vi "TEST - Periodic Trigger.vi"(8 "error in (no error)":errorcluster) -> (0 "error out":errorcluster, 2 "pass":bool)   [LabVIEW 2020]
uses:
  <userlib>/_OpenG.lib/error/error.llb/openg_error.lvlib
  source/library/openg_time.lvlib
panel:
  out "sum":i16
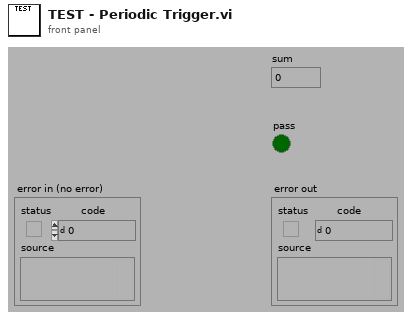
[diagram p1: front panel]
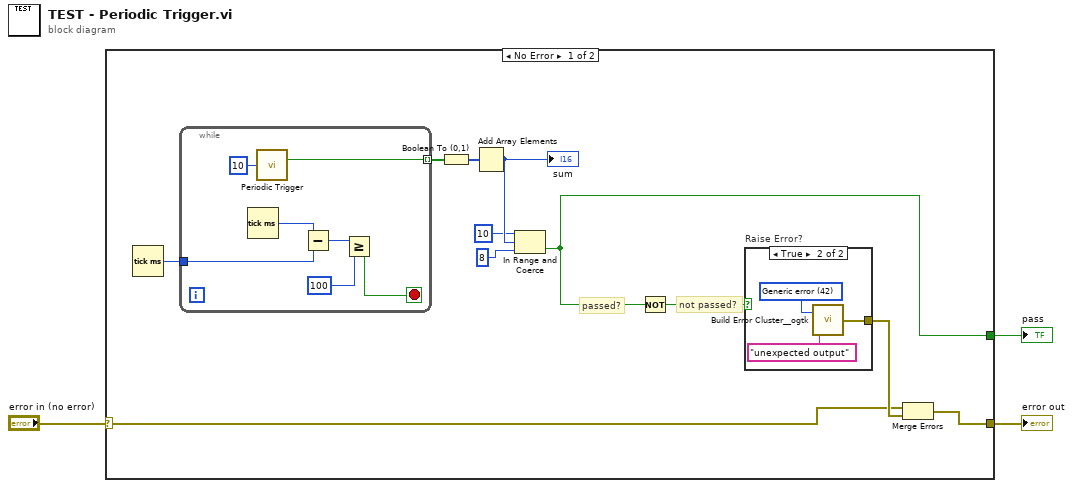
[diagram p0: block diagram]
diagram:
  n1 = case shown="No Error" "error in (no error)" {
    selector: "error in (no error)" -> [w8 w25]
    tunnel: [w4 _] -> w3
    tunnel: [w14 w25] -> w1
    frame No Error {
      # "not passed?"
      # "passed?"
      n2 = Tick Count (ms)() -> (millisecond timer value=w11:u32)
      n3 = while {
        tunnel: w11 -> [w19]
        tunnel: [w20] -> w10 mode=indexing
        stop <- w16 stop-if-true
        n4 = Tick Count (ms)() -> (millisecond timer value=w15:u32)
        n5 = call "Periodic Trigger.vi"("time (ms)"=u32 10) -> ("Triggered"=w20:bool)  [unwired: 12 in, 2 out]
        n6 = Subtract(x=w15, y=w19) -> (x-y=w18:u32)
        n7 = Greater Or Equal?(x=w18, y=u32 100) -> (x >= y?=w16:bool)
      }
      n8 = Boolean To (0,1)(Boolean=w10) -> (0, 1=w9:i16[])
      n9 = Add Array Elements(numeric array=w9) -> (sum=w7:i16)
      "sum" <- w7
      n10 = In Range and Coerce(upper limit=i16 10 ("sum"), x=w7, lower limit=i16 8 ("sum")) -> (In Range?=w4:bool)  [unwired: 1 out]
      n11 = Not(x=w4) -> (.not. x?=w12:bool)
      n12 = case "Raise Error?" shown="True" w12 {
        tunnel: [_ w22] -> w13
        frame False {
        }
        frame True {
          w23 = 42 items=["No error", "Argument error", "Memory is full", "Out of zone", "End of file", "File already open", "Generic file I/O error", "File not found", "File permission error", "Disk is full", "Duplicate path", "Too many files open", "System feature not enabled", "Resource file not found", "Cannot add resource", "Resource not found", "Image not found", "Image memory error", "Pen does not exist", "Config type invalid", "Config token not found", "Config parse error", "Config memory error", "Bad external code format", "Bad external code offset", "External code not present", "Null window", "Destroy window error", "Null menu", "Print aborted", "Bad print record", "Print driver error", "Windows error during printing", "Memory error during printing", "Print dialog error", "Generic print error", "Invalid device refnum", "Device not found", "Device parameter error", "Device unit error", "Cannot open device", "Device call aborted", "Generic error", "Cancelled by user", "Object ID too low", "Object ID too high", "Object not in heap", "Unknown heap", "Unknown object (invalid DefProc)", "Unknown object (DefProc not in table)", "Message out of range", "Invalid (null) method", "Unknown message", "Manager call not supported", "Bad address", "Network operation in progress", "Network operation timed out", "Connection is busy", "Network attribute not supported", "Network error", "Address in use", "System out of memory", "Connection aborted", "Connection refused", "Not connected", "Already connected", "Connection closed", "Initialization error (interapplication manager)", "Bad occurrence", "Wait on unbound occurrence handler", "Occurrence queue overflow", "Datalog type conflict", "Unused", "Unrecognized type (interapplication manager)", "Memory corrupt", "Failed to make temporary DLL", "Old CIN version", "Drag socket not found", "Failed to load drop-object", "Failed to register OLE object", "Failed to release OLE object", "Format specifier type mismatch", "Unknown format specifier", "Too few format specifiers", "Too many format specifiers", "Scan failed", "Newer CIN version", "Error converting to variant", "Runtime menu error", "Password tampered", "Variant attribute not found", "Incompatible variant data type", "Event data is not available", "Event Store is not present", "Occurrence is not found", "Event Queue is not created", "Event info is not available", "Refnum passed is NULL", "Error retrieving Class GUID", "Error retrieving CoClass GUID", "Error retrieving TypeLib GUID.", "Bad built application magic bytes.", "Specific driver is different from the specific driver associated with the Logical Name.", "There is no session opened to the class driver.", "Max Error", "MAX - Error with config objects", "MAX - Error loading configuration", "MAX - Group not supported"]
          n13 = call <userlib>:"Build Error Cluster__ogtk.vi"("String to Prepend to source (\"\")"="unexpected output" ("String to Prepend to source (\"\")"), "code"=w23) -> ("error out"=w22:errorcluster)
        }
      }
      n14 = Merge Errors(w8, w13) -> (w14:errorcluster)
    }
    frame Error {
    }
  }
  "pass" <- w3
  "error out" <- w1
